vi "kvCanUnloadLibrary.vi"(1 "error in (no error)":errorcluster) -> (0 "error out":errorcluster)   [LabVIEW 2023]
doc: "Use this function if you are loading canlib32.dll dynamically (that is, using the Win32 API LoadLibrary) and need to unload it using the Win32 API FreeLibrary. \n\nkvCanUnloadLibrary will free allocated memory, unload the DLLs canlib32.dll has loaded and de-initialize data structures. You must call kvCanInitialize again to use teh API functions in canlib32.dll."
uses:
  canlib32.dll
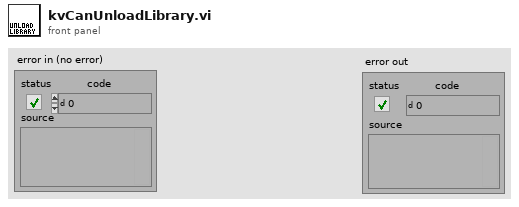
[diagram p1: front panel]
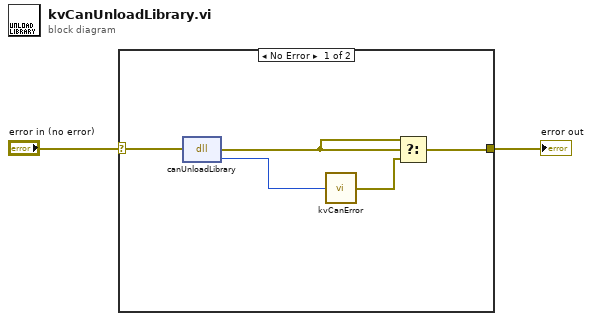
[diagram p0: block diagram]
diagram:
  n1 = case shown="No Error" "error in (no error)" {
    selector: "error in (no error)" -> [w7 w8]
    tunnel: [w3 w8] -> w1
    frame No Error {
      n2 = dll-call lib="canlib32.dll" fn="canUnloadLibrary"(error in=w7) -> (error out=w5:errorcluster, "return type"=w6:i32)  [unwired: 2 in, 1 out]
      n3 = call "kvCanError.vi"("error code"=w6) -> ("error out"=w4:errorcluster)
      n4 = Select(t=w5, s=w5, f=w4) -> (s? t:f=w3:errorcluster)
    }
    frame Error {
    }
  }
  "error out" <- w1
